vi "Gridsearch Visualization.vi"(8 "error in (no error)":errorcluster, 9 "Plot Type":T1 caption="Rate", 10 "Grid parameters":T3={"C start"=-5.0, "C end"=15.0, "C step"=4.0, "Gamma start"=-15.0, "Gamma end"=3.0, "Gamma step"=4.0, "K"=10, "random seed"=-1}, 11 "Confusion matrices":T2[](array[typedef])) -> (0 "error out":errorcluster, 3 "3D Surface Plot":refnum<class "3D Plot Datatype.lvclass">[](array[class]))   [LabVIEW 2014]
uses:
  LibSVM Sparse/Controls/Grid parameters.ctl
  Controls/Binary_ConfusionMatrix.ctl
  <vilib>/Math Plots/3D Math Plots/3D Plot/3D Plot Datatype/3D Plot Datatype.lvclass
  <vilib>/Math Plots/3D Math Plots/3D Surface/3D Surface XCtrl/3D Surface.xctl
  Controls/Plot_Rate.ctl
  <vilib>/Analysis/1siggen.llb/Ramp Pattern by Delta.vi
  <vilib>/gmath/interp.llb/Create Mesh Grid (2D) (x,y arrays).vi
  <vilib>/Math Plots/3D Math Plots/3D Surface/3D Surface Datatype/Public/Plot Helper (Matrix).vi
  <vilib>/Math Plots/3D Math Plots/3D Surface/3D Surface Datatype/3D Surface Datatype.lvclass
  <vilib>/Analysis/NI_AALBase.lvlib
  <vilib>/gmath/NI_Gmath.lvlib
panel:
  out "Graph":refnum<class "3D Plot Datatype.lvclass">[](xcontrol)
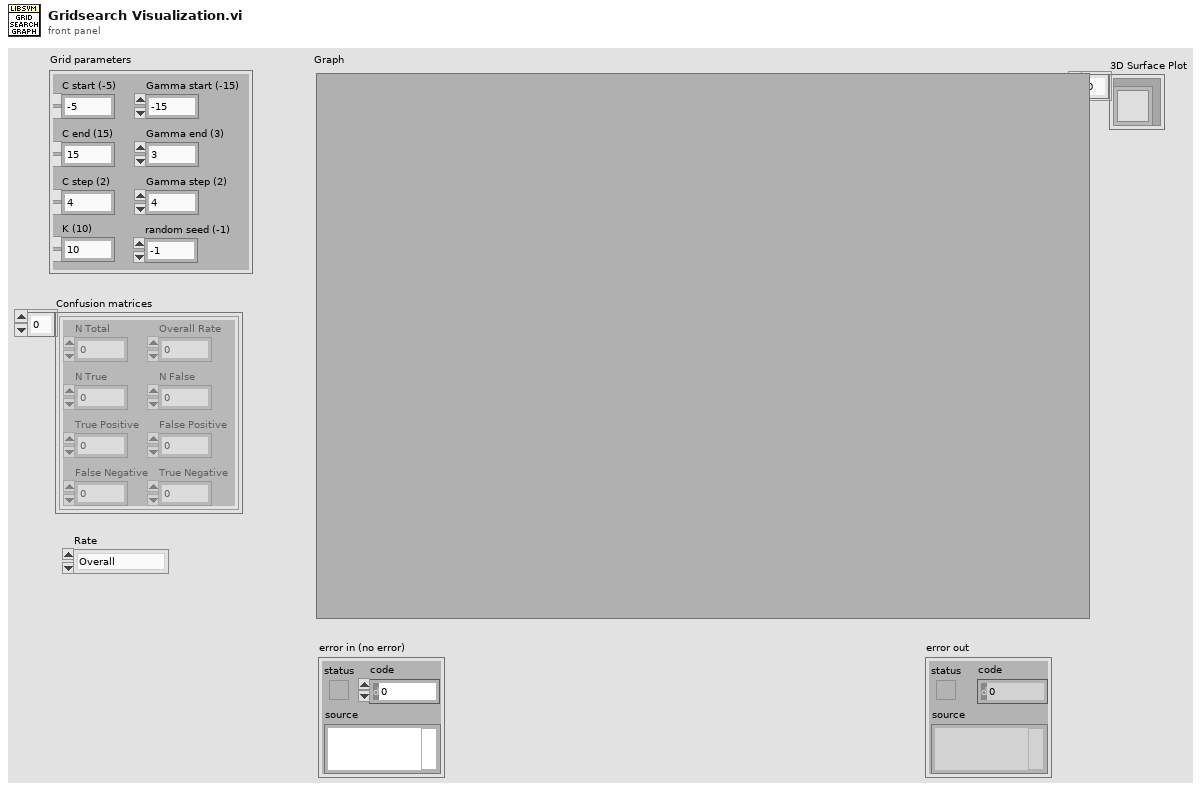
[diagram p1: front panel]
types:
  T1 = typedef "Plot_Rate.ctl" = enum16{"Overall", "Average", "True positive", "True negative", "False positive", "False negative"}
  T2 = typedef "Binary_ConfusionMatrix.ctl" = cluster{"N Total":u32, "N True":u32, "N False":u32, "Overall Rate":dbl, "True Positive":dbl, "False Positive":dbl, "False Negative":dbl, "True Negative":dbl}
  T3 = typedef "Grid parameters.ctl" = cluster{"C start":dbl, "C end":dbl, "C step":dbl, "Gamma start":dbl, "Gamma end":dbl, "Gamma step":dbl, "K":i32, "random seed":i32}
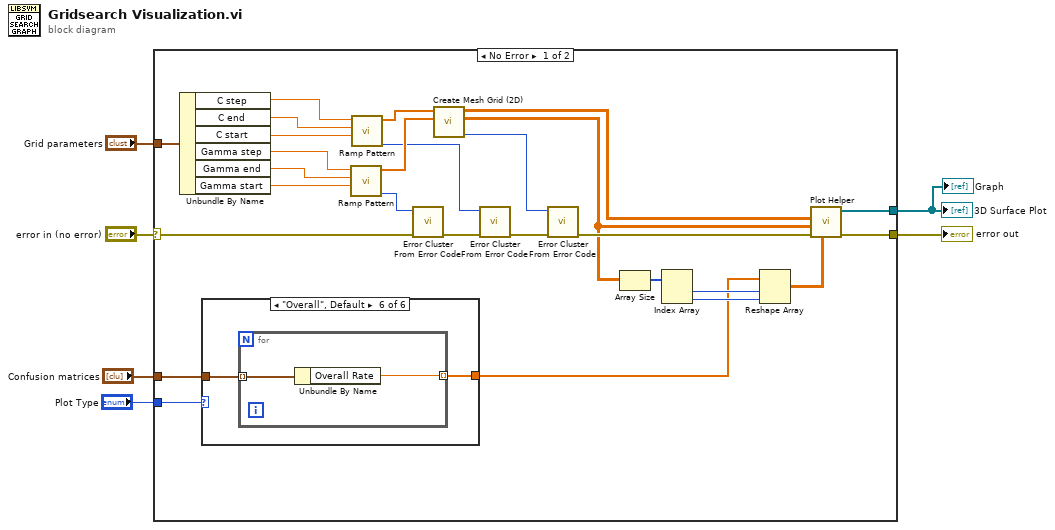
[diagram p0: block diagram]
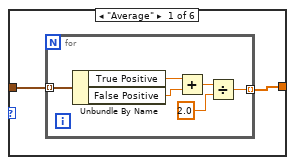
[diagram p2: hidden frame]
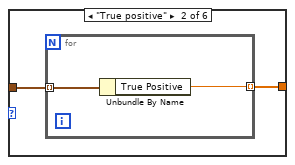
[diagram p3: hidden frame]
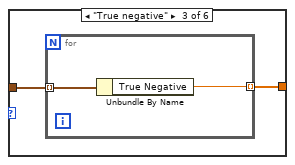
[diagram p4: hidden frame]
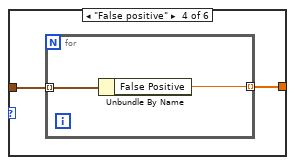
[diagram p5: hidden frame]
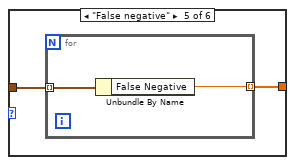
[diagram p6: hidden frame]
diagram:
  n1 = case shown="No Error" "error in (no error)" {
    selector: "error in (no error)" -> [w22 w62]
    tunnel: [w33 w62] -> w6
    tunnel: [w32 _] -> w4
    tunnel: "Confusion matrices" -> [w13 _]
    tunnel: "Grid parameters" -> [w29 _]
    tunnel: "Plot Type" -> [w12 _]
    frame No Error {
      n2 = Unbundle By Name(w29) -> ("C step"=w28:dbl, "C end"=w27:dbl, "C start"=w26:dbl, "Gamma step"=w25:dbl, "Gamma end"=w24:dbl, "Gamma start"=w23:dbl)
      n3 = case shown="\"Overall\", Default" w12 {
        tunnel: w13 -> [w35 w43 w47 w51 w55 w59]
        tunnel: [w34 w42 w46 w50 w54 w58] -> w9
        frame "Average" {
          n4 = for {
            tunnel: w35 -> [w41] mode=indexing
            tunnel: [w36] -> w34 mode=indexing
            n5 = Unbundle By Name(w41) -> ("True Positive"=w40:dbl, "False Positive"=w39:dbl)
            n6 = Add(x=w40, y=w39) -> (x+y=w38:dbl)
            n7 = Divide(x=w38, y=2.0) -> (x/y=w36:dbl)
          }
        }
        frame "True positive" {
          n8 = for {
            tunnel: w43 -> [w45] mode=indexing
            tunnel: [w44] -> w42 mode=indexing
            n9 = Unbundle By Name(w45) -> ("True Positive"=w44:dbl)
          }
        }
        frame "True negative" {
          n10 = for {
            tunnel: w47 -> [w49] mode=indexing
            tunnel: [w48] -> w46 mode=indexing
            n11 = Unbundle By Name(w49) -> ("True Negative"=w48:dbl)
          }
        }
        frame "False positive" {
          n12 = for {
            tunnel: w51 -> [w53] mode=indexing
            tunnel: [w52] -> w50 mode=indexing
            n13 = Unbundle By Name(w53) -> ("False Positive"=w52:dbl)
          }
        }
        frame "False negative" {
          n14 = for {
            tunnel: w55 -> [w57] mode=indexing
            tunnel: [w56] -> w54 mode=indexing
            n15 = Unbundle By Name(w57) -> ("False Negative"=w56:dbl)
          }
        }
        frame "Overall", Default {
          n16 = for {
            tunnel: w59 -> [w61] mode=indexing
            tunnel: [w60] -> w58 mode=indexing
            n17 = Unbundle By Name(w61) -> ("Overall Rate"=w60:dbl)
          }
        }
      }
      n18 = call-poly <vilib>:"Ramp Pattern.vi"("start"=w23, "end"=w24, "delta"=w25) -> ("error"=w21:i32, "Ramp Pattern"=w30:dbl[])  [unwired: 6 in, 1 out]
      n19 = call-poly <vilib>:"Ramp Pattern.vi"("start"=w26, "end"=w27, "delta"=w28) -> ("error"=w19:i32, "Ramp Pattern"=w31:dbl[])  [unwired: 6 in, 1 out]
      n20 = call <vilib>:"Error Cluster From Error Code.vi"("error in (no error)"=w22, "error code (0)"=w21) -> ("error out"=w20:errorcluster)  [unwired: 7 in]
      n21 = call-poly <vilib>:"Create Mesh Grid (2D).vi"("y domain"=w30, "x domain"=w31) -> ("error"=w17:i32, "Y"=w7:dbl[][], "X"=w14:dbl[][])  [unwired: 7 in]
      n22 = call <vilib>:"Error Cluster From Error Code.vi"("error in (no error)"=w20, "error code (0)"=w19) -> ("error out"=w18:errorcluster)  [unwired: 7 in]
      n23 = call <vilib>:"Error Cluster From Error Code.vi"("error in (no error)"=w18, "error code (0)"=w17) -> ("error out"=w16:errorcluster)  [unwired: 7 in]
      n24 = Array Size(array=w7) -> (size(s)=w15:i32[])
      n25 = Index Array(array=w15) -> (element #1=w11:i32, element #2=w10:i32)  [unwired: 2 in]
      n26 = Reshape Array(w9, w11, w10) -> (w8:dbl[][])
      n27 = call-poly <vilib>:"Plot Helper.vi"("z matrix"=w8, "error in (no error)"=w16, "y matrix"=w7, "x matrix"=w14) -> ("error out"=w33:errorcluster, "3D Plot lvclass Array out"=w32:refnum<class "3D Plot Datatype.lvclass">[])  [unwired: 2 in, 4 out]
    }
    frame Error {
    }
  }
  "error out" <- w6
  "3D Surface Plot" <- w4
  "Graph" <- w4
